vi "Flatten Value.vi"(8 "Error In":errorcluster, 11 "2D Bool In":refnum<class "2D Bool.lvclass">) -> (0 "Error Out":errorcluster, 1 "Value":string, 3 "2D Bool Out":refnum<class "2D Bool.lvclass">)   [LabVIEW 2017, in "Tree API.lvlib" / "2D Bool.lvclass"]
doc: "Dynamic dispatch interface for flattening Tree Data classes to string."
uses:
  2D Bool.lvclass
  Tree Manager/Tree.lvclass
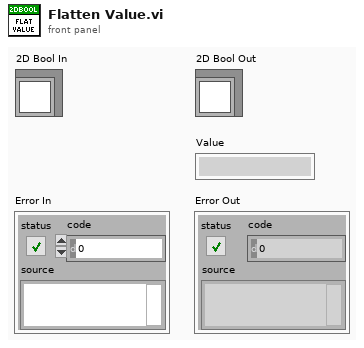
[diagram p1: front panel]
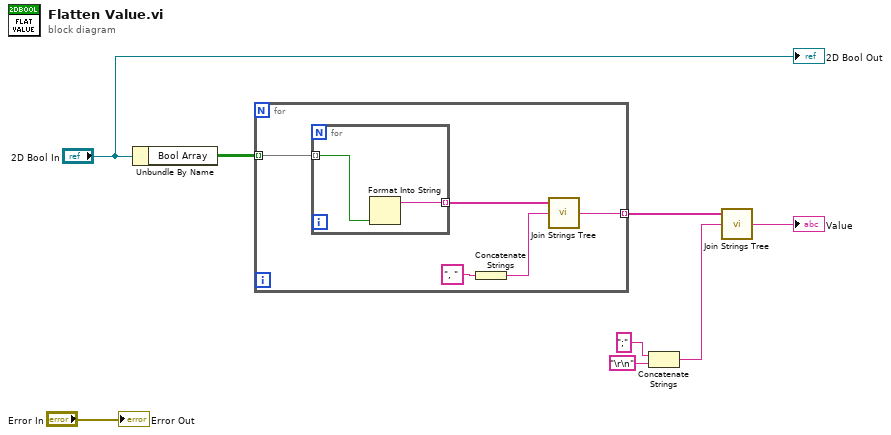
[diagram p0: block diagram]
diagram:
  n1 = Unbundle By Name("2D Bool In") -> ("Bool Array"=w8:bool[][])
  n2 = for {
    tunnel: w8 -> [w13] mode=indexing
    tunnel: [w11] -> w7 mode=indexing
    n3 = for {
      tunnel: w13 -> [w15] mode=indexing
      tunnel: [w14] -> w12 mode=indexing
      n4 = Format Into String(w15) -> (resulting string=w14:string)  [unwired: 3 in, 1 out]
    }
    n5 = Concatenate Strings(", " ("Separator (,)")) -> (w9:string)
    n6 = call "Join Strings Tree.vi"("Separator (,)"=w9, "Strings In"=w12) -> ("String"=w11:string)  [unwired: 1 in]
  }
  n7 = Concatenate Strings(";" ("Separator (,)"), "\r\n") -> (w3:string)
  n8 = call "Join Strings Tree.vi"("Separator (,)"=w3, "Strings In"=w7) -> ("String"=→"Value":string)  [unwired: 1 in]
  "2D Bool Out" <- "2D Bool In"
  "Error Out" <- "Error In"
